vi "epxMAUpdate1bitword.vi"(6 "input valid":bool=TRUE, 8 "expFactor":i16=-8, 9 "min delta":fxp<+,12,-14>, 10 "update":fxp<+/-,24,1>, 11 "carryIn":fxp<+/-,28,2>) -> (0 "output valid":bool, 3 "carryOut":fxp<+/-,28,2>)   [LabVIEW 2016]
uses:
  <vilib>/rvi/FXPMathLib/FxpSub/XNode/nifxpmath_Sub.xnode
  <vilib>/rvi/FXPMathLib/FxpAdd/XNode/nifxpmath_Add.xnode
  <vilib>/rvi/FXPMathLib/sim/FxpSim.dll
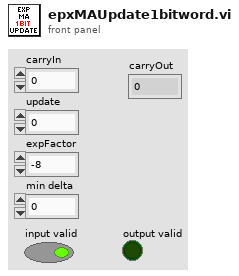
[diagram p1: front panel]
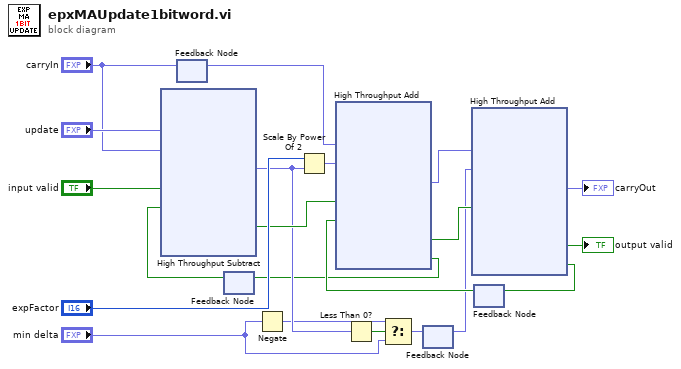
[diagram p0: block diagram]
diagram:
  n1 = feedback #1() -> (w17:fxp<+/-,28,2>)  [unwired: 1 in]
  n2 = feedback-in #1("carryIn") -> ()
  n3 = feedback #2() -> (w2:bool)  [unwired: 1 in]
  n4 = xnode "High Throughput Subtract"("x"="update", "y"="carryIn", "input valid"="input valid", "ready for output (T)"=w2) -> ("x-y"=w7:fxp<+/-,28,2>, "output valid"=w13:bool)  [unwired: 1 out]
  n5 = Negate(x="min delta") -> (-x=w5:fxp<+/-,12,-14>)
  n6 = Scale By Power Of 2(n="expFactor", x=w7) -> (x*2^n=w14:fxp<+/-,28,2>)
  n7 = Less Than 0?(x=w7) -> (x < 0?=w6:bool)
  n8 = Select(t=w5, s=w6, f="min delta") -> (s? t:f=w8:fxp<+/-,13,-13>)
  n9 = feedback #3() -> (w9:fxp<+/-,13,-13>)  [unwired: 1 in]
  n10 = feedback-in #3(w8) -> ()
  n11 = feedback #4() -> (w12:bool)  [unwired: 1 in]
  n12 = xnode ("High Throughput Add")("x"=w17, "y"=w14, "input valid"=w13, "ready for output (T)"=w12) -> ("x+y"=w10:fxp<+/-,28,2>, "output valid"=w11:bool, "ready for input"=w3:bool)
  n13 = feedback-in #2(w3) -> ()
  n14 = xnode ("High Throughput Add")("x"=w10, "y"=w9, "input valid"=w11) -> ("x+y"=→"carryOut":fxp<+/-,28,2>, "output valid"=→"output valid":bool, "ready for input"=w20:bool)  [unwired: 1 in]
  n15 = feedback-in #4(w20) -> ()
